vi "GUI_TRA_Staging.vi"() -> ()   [LabVIEW 2013]
uses:
  <vilib>/Utility/file.llb/Write To Spreadsheet File (DBL).vi
  <vilib>/Utility/file.llb/Write To Spreadsheet File (string).vi
  Device Drivers/TRAServer/HomingType_TypDef.ctl
  Device Drivers/TRAServer/TRAServer.lvclass
  Device Drivers/TRAServer/StatusTRA_TypDef.ctl
  Device Drivers/shared/OnOffTypeDef.ctl
panel:
  in  "Multicolumn Listbox 2":refnum<vi>
  in  "Main Tap 2":refnum<vi>
  out "all pos array":refnum<vi>[][](array[refnum])
  out "all status array":refnum<vi>[][](array[refnum])
  out "indecator ref array 2":refnum<vi>[](array[refnum])
  out "indecator ref array":refnum<vi>[](array[refnum])
  in  "time to wait (TCP) 2":i32=10
  in  "plot":bool=TRUE
  out "ratio(h)":bool
  out "fixsize":bool
  out "error (h)":bool
  out "Device Name (h)":string="StagingTRA1"
  in  "Main Tap":T1(tab)
  in  "stepSize":dbl=0.01
  in  "Status":T2=enum."DISABLE" caption="Status Y"
  in  "Up":bool
  in  "Down":bool
  in  "Right":bool
  in  "Left":bool
  in  "Status":T2=enum."DISABLE" caption="Status X"
  in  "Position":dbl caption="X" format="%#_12g"
  in  "Position":dbl caption="Y" format="%#_12g"
  in  "Mirror":T3(ring)=enum."DiagStage"
  in  "device status":string="Initialized"
  in  "Home 3":bool
  in  "Home 2":bool
  out "Status.Axis 6":T2=enum."DISABLE" caption="Status X"
  out "Status.Axis 5":T2=enum."DISABLE" caption="Status X"
  out "Status.Axis 4":T2=enum."DISABLE" caption="Status X"
  out "Status.Axis 3":T2=enum."DISABLE" caption="Status X"
  out "Status.Axis 2":T2=enum."DISABLE" caption="Status X"
  out "Status.Axis 1":T2=enum."DISABLE" caption="Status X"
  out "Status.Axis 1":T2=enum."DISABLE" caption="Status X"
  out "Status.Axis 2":T2=enum."DISABLE" caption="Status X"
  out "Status.Axis 3":T2=enum."DISABLE" caption="Status X"
  out "Status.Axis 4":T2=enum."DISABLE" caption="Status X"
  out "Status.Axis 5":T2=enum."DISABLE" caption="Status X"
  out "Status.Axis 6":T2=enum."DISABLE" caption="Status X"
  out "Status.Axis 7":T2=enum."DISABLE" caption="Status X"
  out "Status.Axis 8":T2=enum."DISABLE" caption="Status X"
  out "Status.Axis 9":T2=enum."DISABLE" caption="Status X"
  out "Status.Axis 10":T2=enum."DISABLE" caption="Status X"
  out "Status.Axis 11":T2=enum."DISABLE" caption="Status X"
  out "Status.Axis 12":T2=enum."DISABLE" caption="Status X"
  in  "Home 1":bool
  in  "Path":path
  in  "Save":bool
  in  "Multicolumn Listbox":i32(listbox)
  in  "Position.Axis 1":dbl=3.05 caption="X"
  in  "Position.Axis 2":dbl=3.05 caption="Y"
  in  "Position.Axis 4":dbl=3.05 caption="X"
  in  "Position.Axis 3":dbl=3.05 caption="Y"
  in  "Position.Axis 6":dbl=3.05 caption="X"
  in  "Position.Axis 5":dbl=3.05 caption="Y"
  in  "Position.Axis 18":dbl=3.05 caption="X"
  in  "Position.Axis 17":dbl=3.05 caption="Y"
  in  "Position.Axis 16":dbl=3.05 caption="X"
  in  "Position.Axis 15":dbl=3.05 caption="Y"
  in  "Position.Axis 14":dbl=3.05 caption="X"
  in  "Position.Axis 13":dbl=3.05 caption="Y"
  in  "Position.Axis 12":dbl=3.05 caption="X"
  in  "Position.Axis 11":dbl=3.05 caption="Y"
  in  "Position.Axis 10":dbl=3.05 caption="X"
  in  "Position.Axis 9":dbl=3.05 caption="Y"
  in  "Position.Axis 8":dbl=3.05 caption="Y"
  in  "Position.Axis 7":dbl=3.05 caption="X"
  in  "take images":bool
  out "appended array 4":cluster{dbl[], dbl[]}[](graph)
  in  "Boolean":bool
  in  "path":path=path "I:/project/Staging/TRAMotors/temp"
  out "centerY":dbl=547.3047962900782
  out "centerX":dbl=832.2888350246396
  in  "backlash":dbl
  in  "backlash 2":dbl
  out "local Port":u16=65435
  in  "timeout ms (slow resp)":i32=500
  in  "reset":bool
  out "image con closed":bool
  out "image \nconnection":bool
  out "image con closed 2":bool
  out "All Devices (h)":string[](array[string])=["StagingTRA1"]
  out "Remote Host":string="192.168.11.97"
  out "port or service name":u16=65434
  out "port or service name out":u16=65400
  in  "time to wait (TCP)":i32=10
  out "error out":errorcluster
  out "connections (hidden)":variant[](array[variant])=[variant(refnum<k16> refnum), variant(refnum<k16> refnum)]
  in  "time to wait (main loop)":i32=10
  out "Data String":string="Status.Axis 1,DISABLE\r\nStatus.Axis 2,DISABLE\r\nStatus.Axis 3,NOT REFERENCED\r\nStatus.Axis 4,NOT REFERENCED\r\nStatus.Axis 5,DISABLE\r\nStatus.Axis 6,NOT REFERENCED\r\nPosition.Axis 1,3.779970\r\nPosition.Axis 2,2.684000\r\nPosition.Axis 3,-0.000000\r\nPosition.Axis 4,-0.000000\r\nPosition.Axis 5,0.000000\r\nPosition.Axis 6,39.383880\r\nDisable.Axis 1,on\r\nDisable.Axis 2,on\r\nDisable.Axis 3,on\r\nDisable.Axis 4,on\r\nDisable.Axis 5,on\r\nDisable.Axis 6,on\r\nHomingType.Axis 1,EoR- switch only\r\nHomingType.Axis 2,EoR- switch only\r\nHomingType.Axis 3,EoR- switch only\r\nHomingType.Axis 4,EoR- switch only\r\nHomingType.Axis 5,MZ switch only\r\nHomingType.Axis 6,EoR- switch only\r\nHome.Axis 1,off\r\nHome.Axis 2,off\r\nHome.Axis 3,off\r\nHome.Axis 4,off\r\nHome.Axis 5,off\r\nHome.Axis 6,off\r\nLimits.pos.Axis 1,6.000000\r\nLimits.pos.Axis 2,6.000000\r\nLimits.pos.Axis 3,6.000000\r\nLimits.pos.Axis 4,6.000000\r\nLimits.pos.Axis 5,51.000000\r\nLimits.pos.Axis 6,6.000000\r\nLimits.neg.Axis 1,0.000000\r\nLimits.neg.Axis 2,0.000000\r\nLimits.neg.Axis 3,0.000000\r\nLimits.neg.Axis 4,0.000000\r\nLimits.neg.Axis 5,-49.000000\r\nLimits.neg.Axis 6,0.000000\r\nbacklash.Axis 1,\r\nbacklash.Axis 2,\r\nbacklash.Axis 3,\r\nbacklash.Axis 4,\r\nbacklash.Axis 5,\r\nbacklash.Axis 6,\r\ndevice status,Initialized\r\n"
  in  "Local Saving Path":path
  out "Nr.":i32=2
  out "error (h) 2":bool
  in  "shotnumber":i32
  out "String":string="wait>>Status.Axis 1,Status.Axis 2,Status.Axis 3,Status.Axis 4,Status.Axis 5,Status.Axis 6,Position.Axis 1,Position.Axis 2,Position.Axis 3,Position.Axis 4,Position.Axis 5,Position.Axis 6,Disable.Axis 1,Disable.Axis 2,Disable.Axis 3,Disable.Axis 4,Disable.Axis 5,Disable.Axis 6,HomingType.Axis 1,HomingType.Axis 2,HomingType.Axis 3,HomingType.Axis 4,HomingType.Axis 5,HomingType.Axis 6,Home.Axis 1,Home.Axis 2,Home.Axis 3,Home.Axis 4,Home.Axis 5,Home.Axis 6,Limits.pos.Axis 1,Limits.pos.Axis 2,Limits.pos.Axis 3,Limits.pos.Axis 4,Limits.pos.Axis 5,Limits.pos.Axis 6,Limits.neg.Axis 1,Limits.neg.Axis 2,Limits.neg.Axis 3,Limits.neg.Axis 4,Limits.neg.Axis 5,Limits.neg.Axis 6,TargetPos.Axis 1,TargetPos.Axis 2,TargetPos.Axis 3,TargetPos.Axis 4,TargetPos.Axis 5,TargetPos.Axis 6,backlash.Axis 1,backlash.Axis 2,backlash.Axis 3,backlash.Axis 4,backlash.Axis 5,backlash.Axis 6,device status"
  in  "Limits.pos":dbl=51.0
  in  "Home":T4
  in  "Disable":T4=enum."on"
  in  "HomingType":T5=enum."MZ switch only"
  in  "Disable":T4=enum."on"
  in  "HomingType":T5=enum."MZ switch only"
  in  "Home":T4
  in  "Limits.pos":dbl=51.0
  in  "Limits.neg":dbl=-49.0
  in  "Limits.neg":dbl=-49.0
  in  "Mirror 2":T3(ring)
  out "error message":string
  out "Data Connection out":bool=TRUE
  # "Position"
  # "Chassi 1"
  # "Chassi 2"
  # "Chassi 3"
  # "X"
  # "Y"
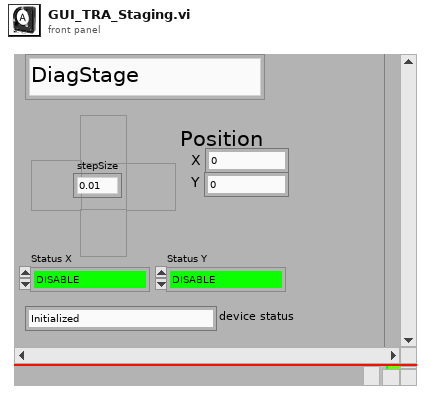
[diagram p1: front panel]
types:
  T1 = enum32{"Main", "Status", "Position", "Position 2", "Temp", "Network", "Internal", "MotorSettings"}
  T2 = typedef "TRAServer.lvclass/StatusTRA_TypDef.ctl" = enum16{"NOT REFERENCED", "CONFIGURATION", "HOMING", "MOVING", "READY", "DISABLE", "JOGGING"}
  T3 = enum16{"M1", "BS", "M3", "OAP1", "M4", "OAP2", "M5", "DiagStage", "SIM"}
  T4 = typedef "OnOffTypeDef.ctl" = enum16{"off", "on"}
  T5 = typedef "TRAServer.lvclass/HomingType_TypDef.ctl" = enum16{"MZ switch and encoder Index", "current position as HOME", "MZ switch only", "EoR- switch and encoder Index", "EoR- switch only"}
  T6 = cluster{"Chassi Nr":i32, "X":string, "Y":string, "name":string}[]
  T7 = cluster{"Chassi Nr":i32, "X":string, "Y":string, "name":string}
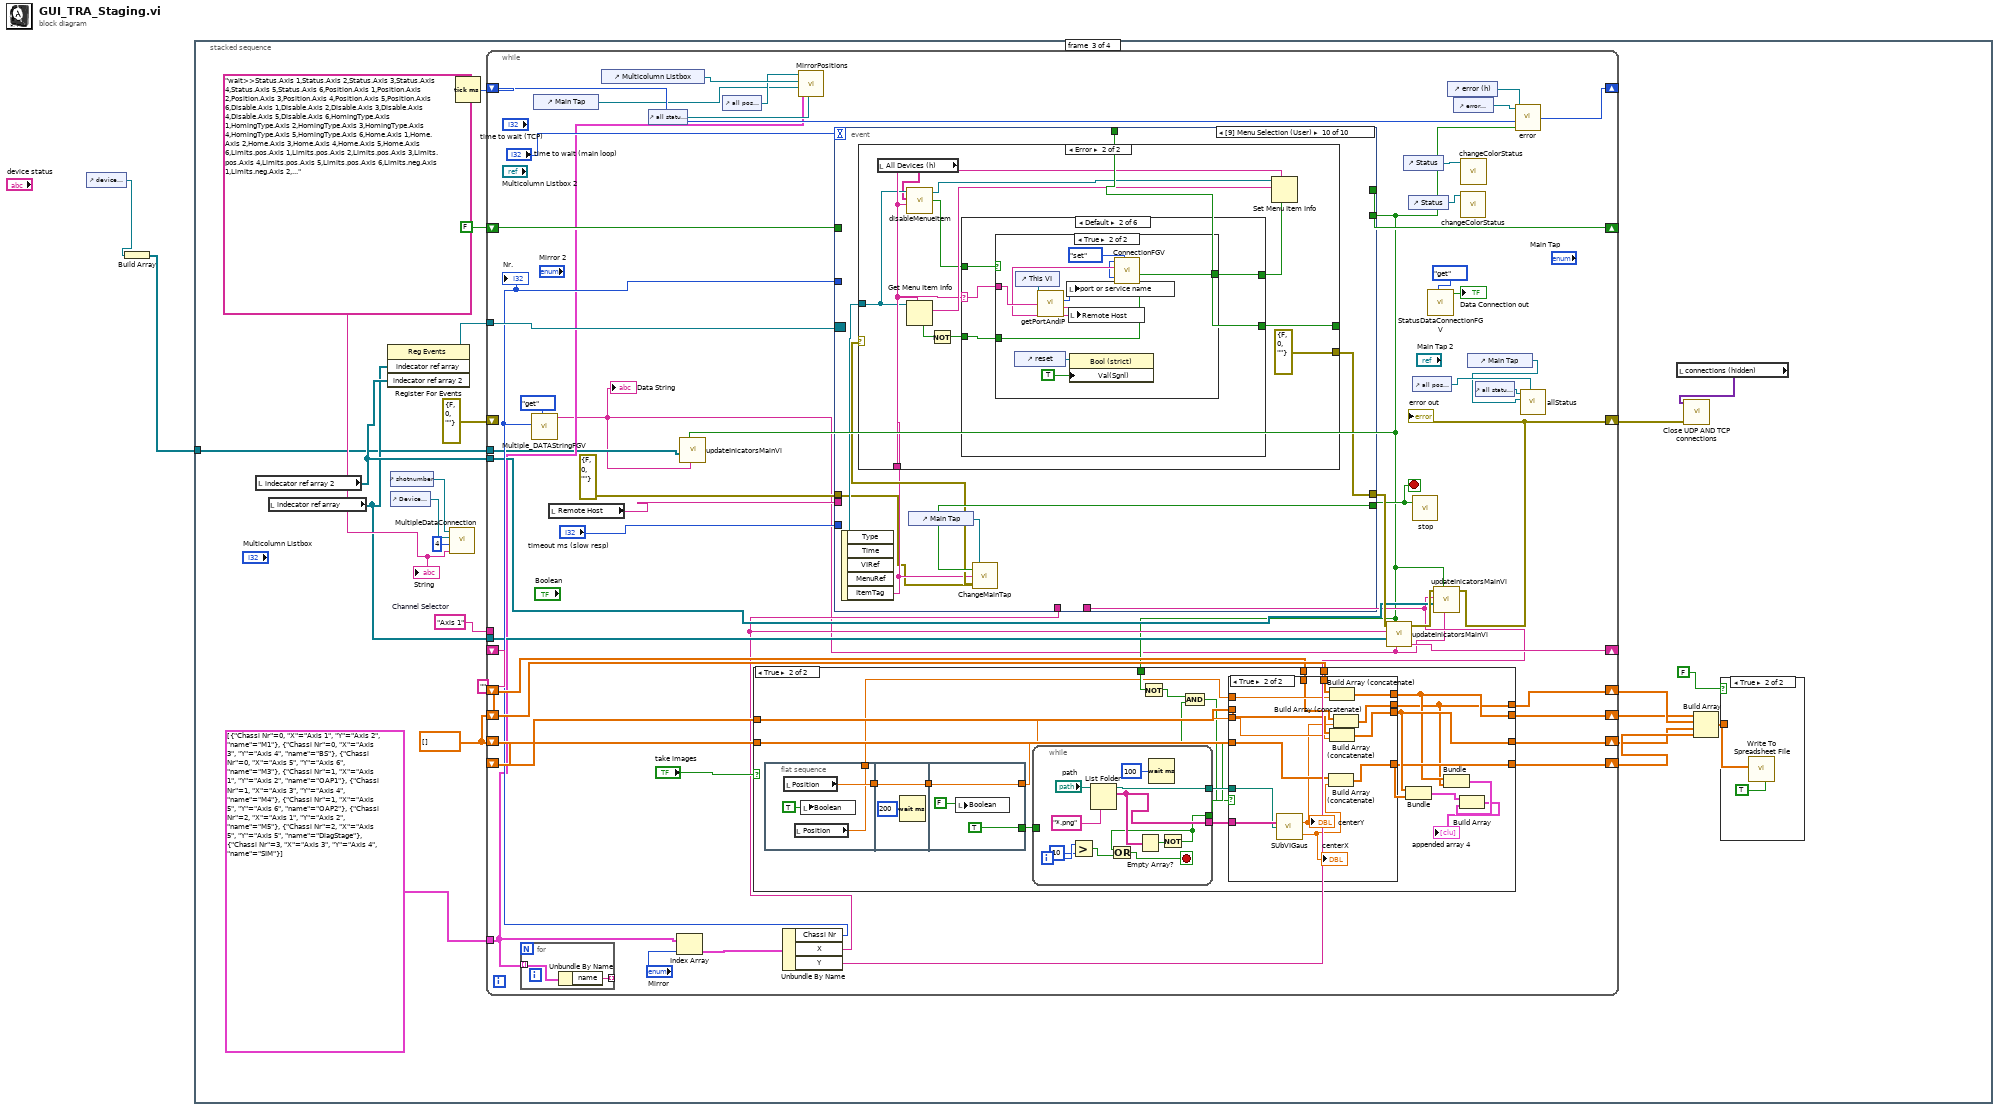
[diagram p0: block diagram]
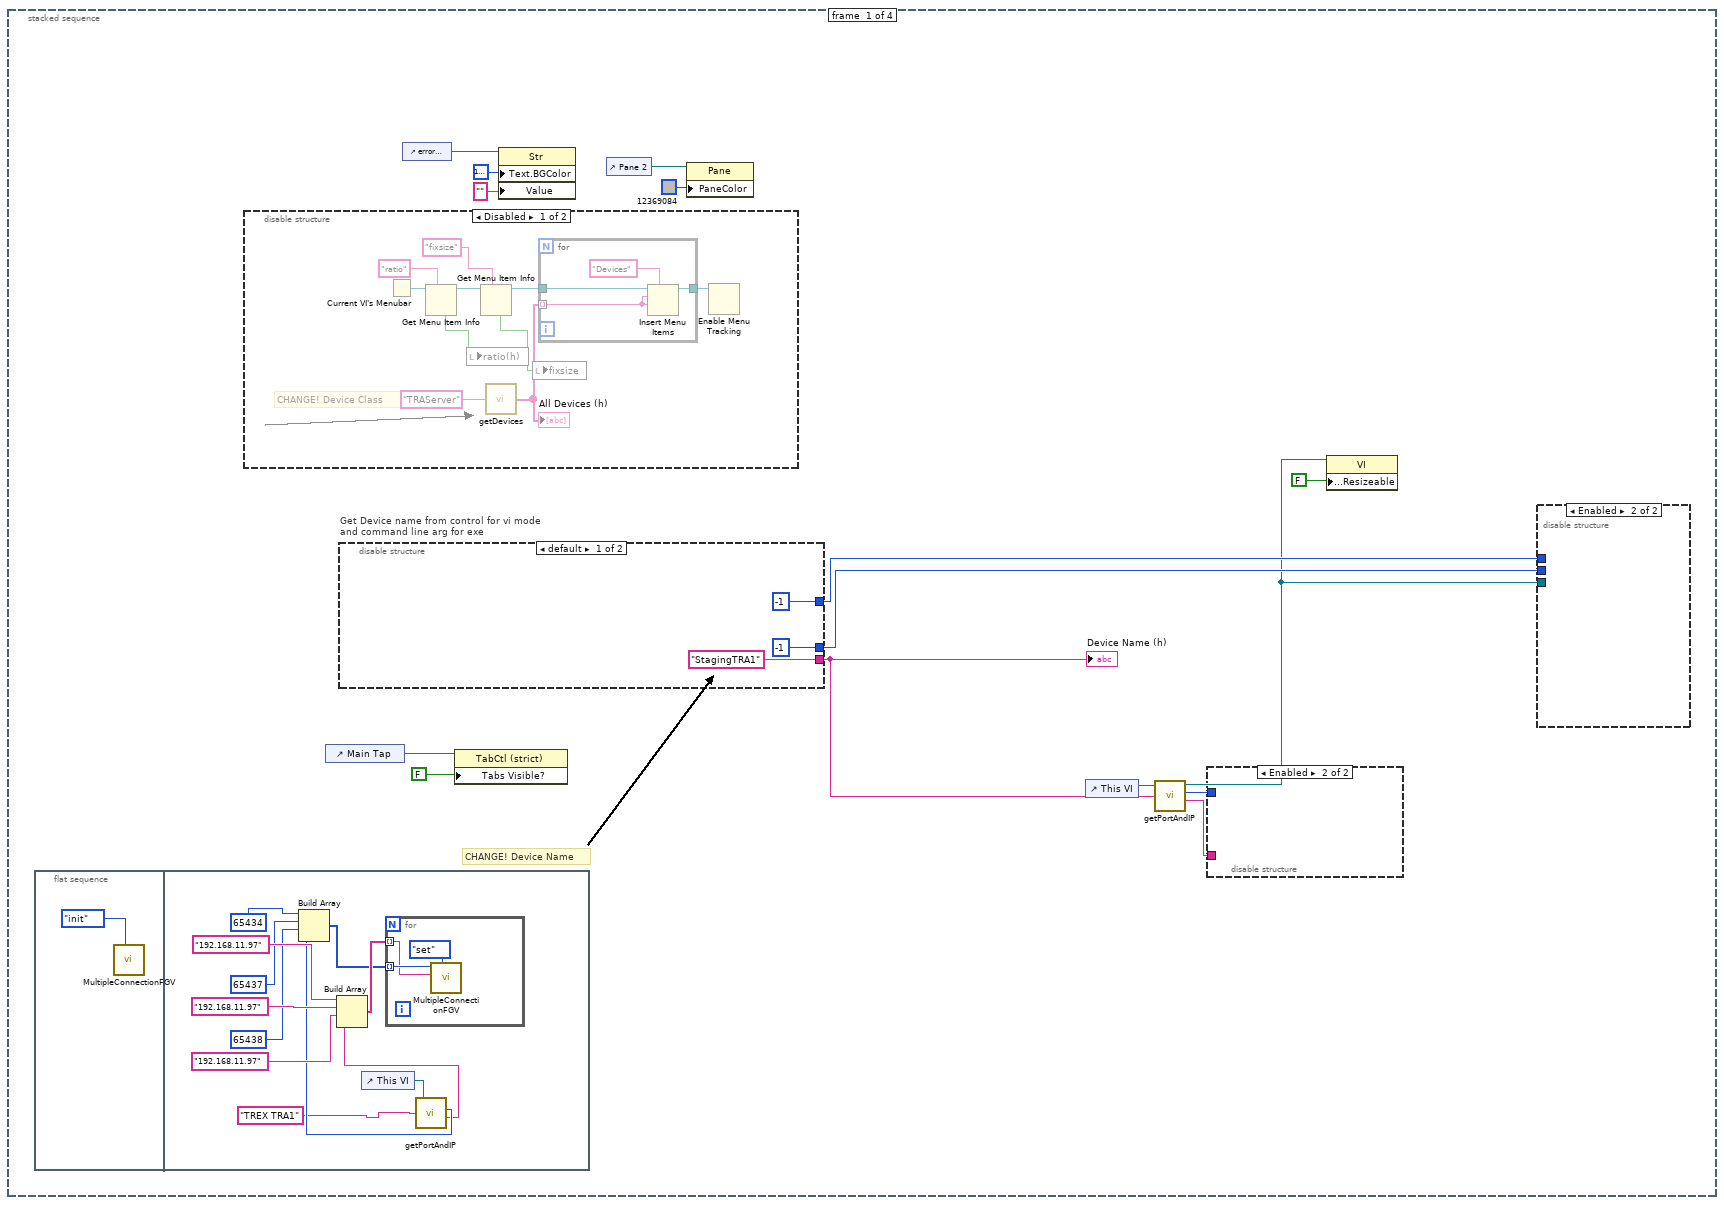
[diagram p2: hidden frame]
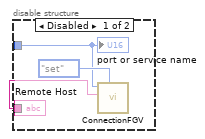
[diagram p4: hidden frame]
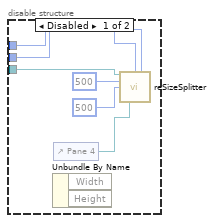
[diagram p5: hidden frame]
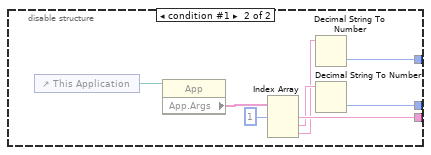
[diagram p6: hidden frame]
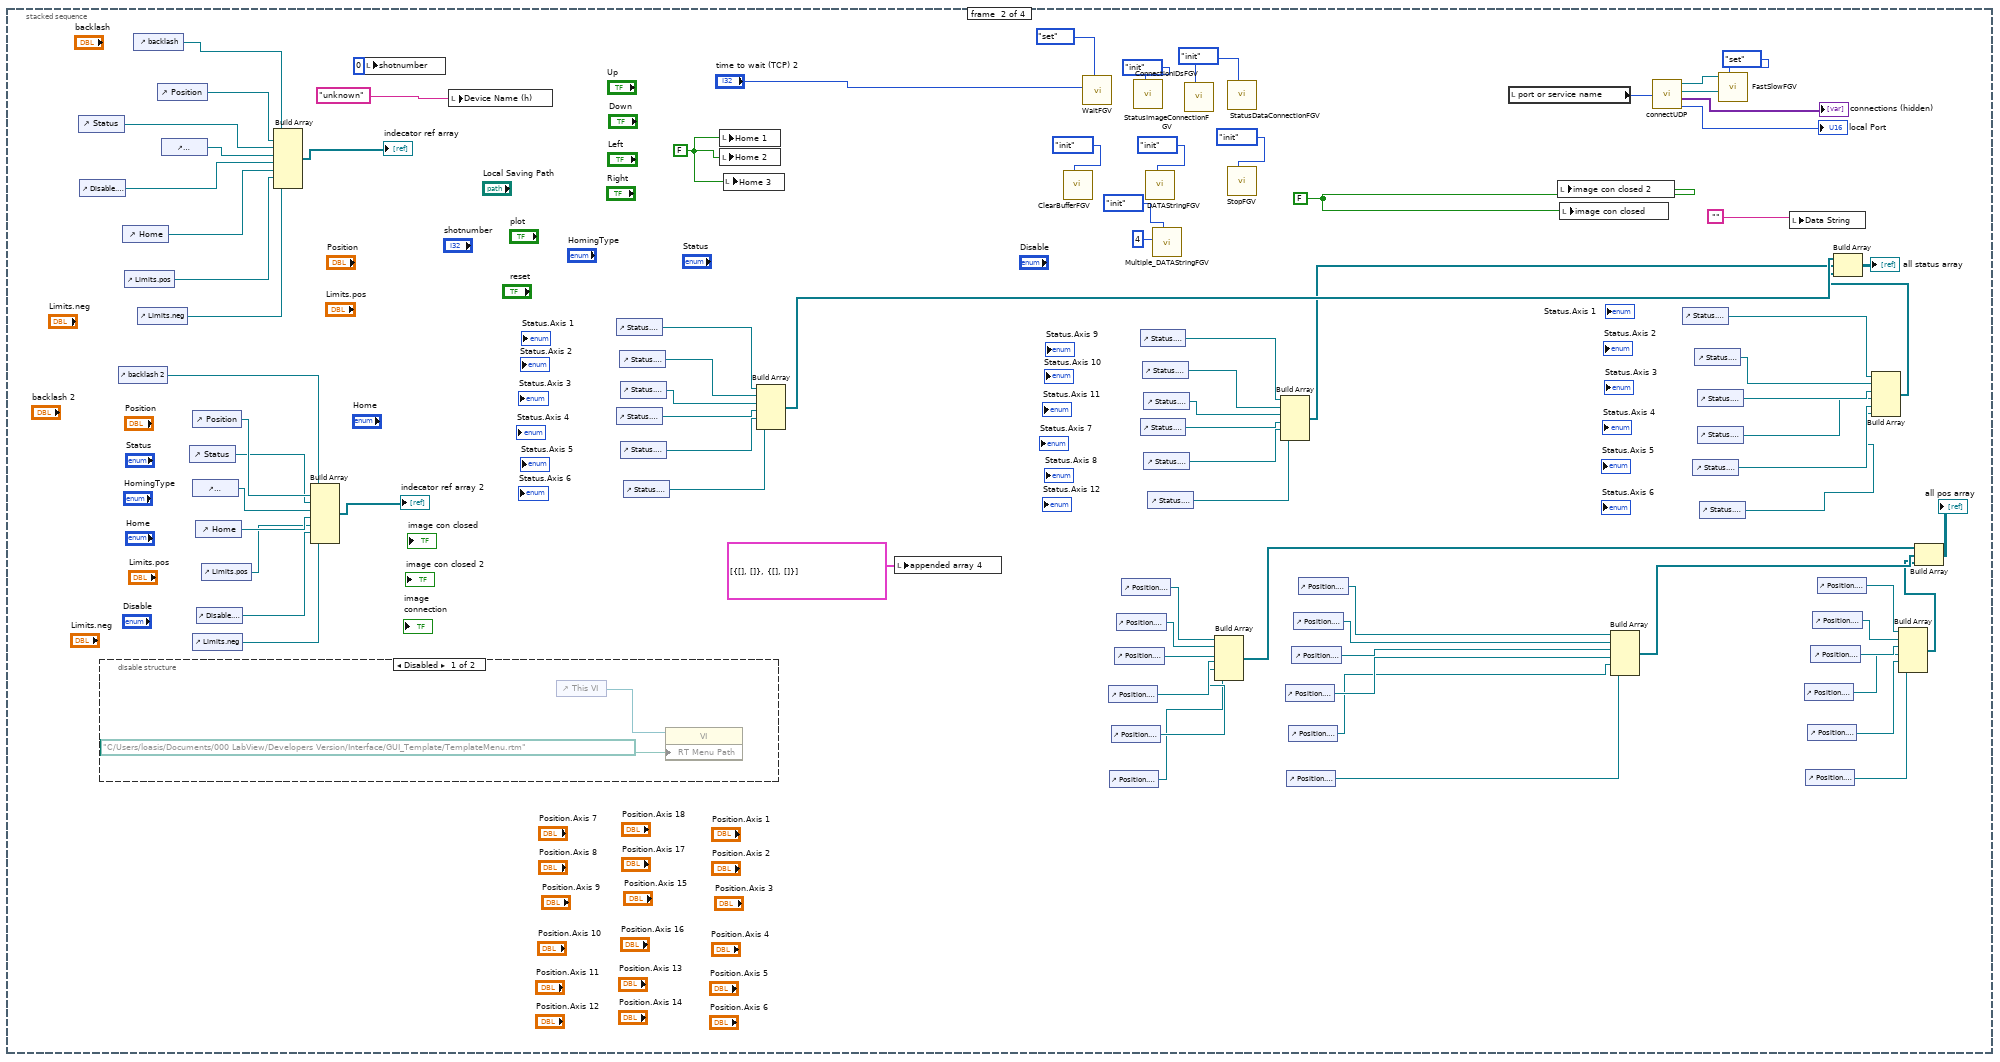
[diagram p7: hidden frame]
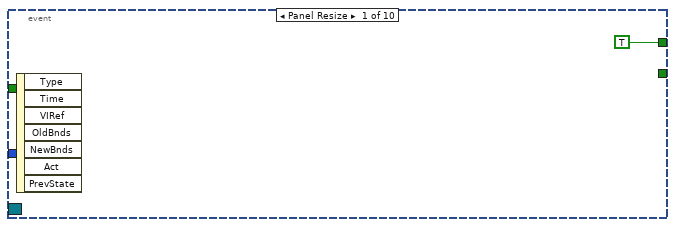
[diagram p12: hidden frame]
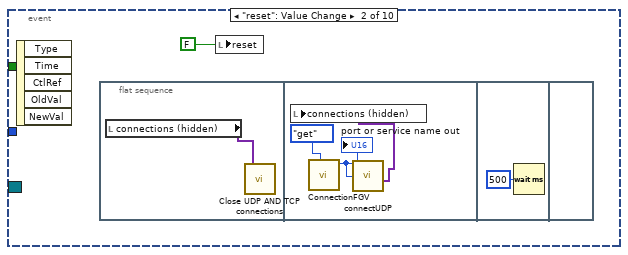
[diagram p13: hidden frame]
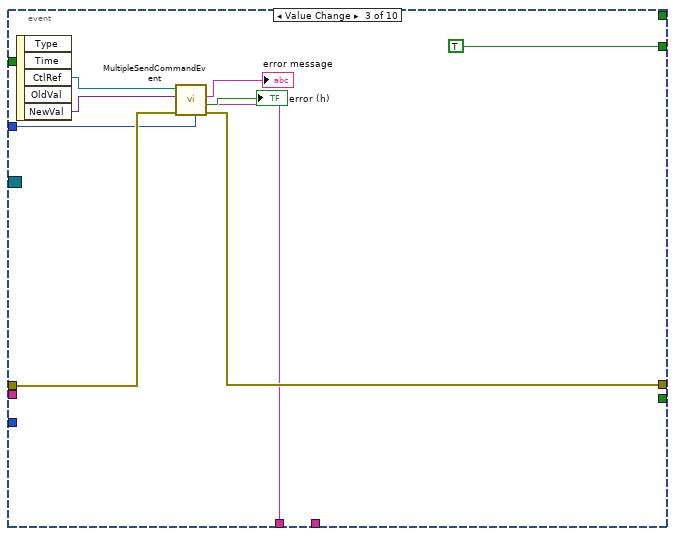
[diagram p14: hidden frame]
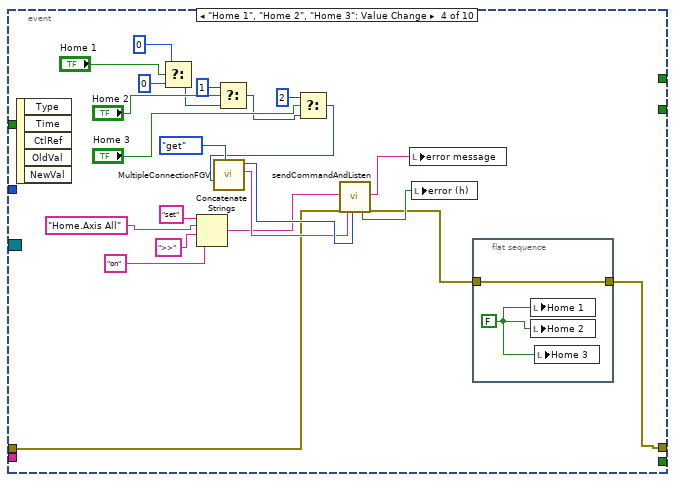
[diagram p15: hidden frame]
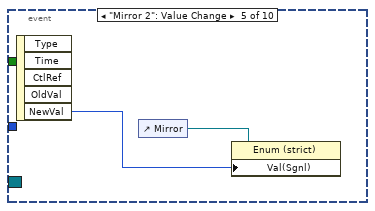
[diagram p16: hidden frame]
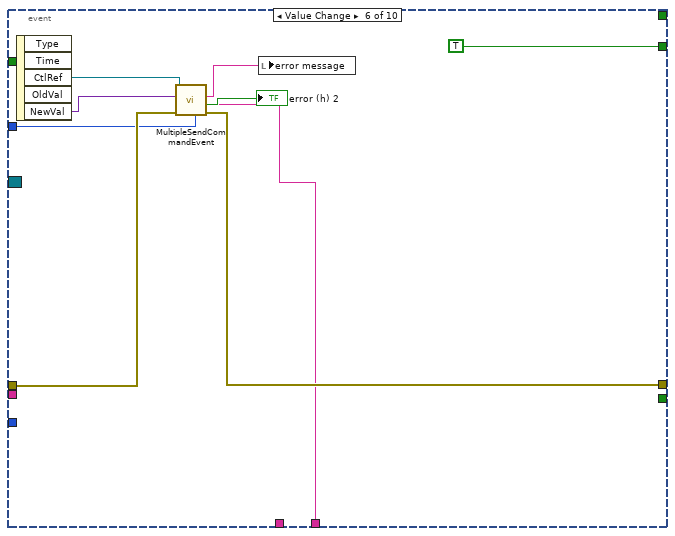
[diagram p17: hidden frame]
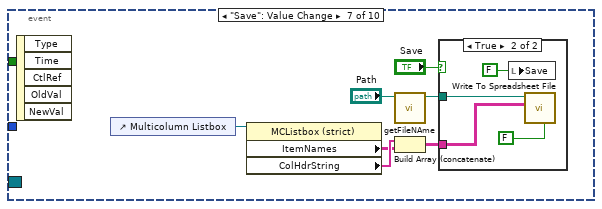
[diagram p18: hidden frame]
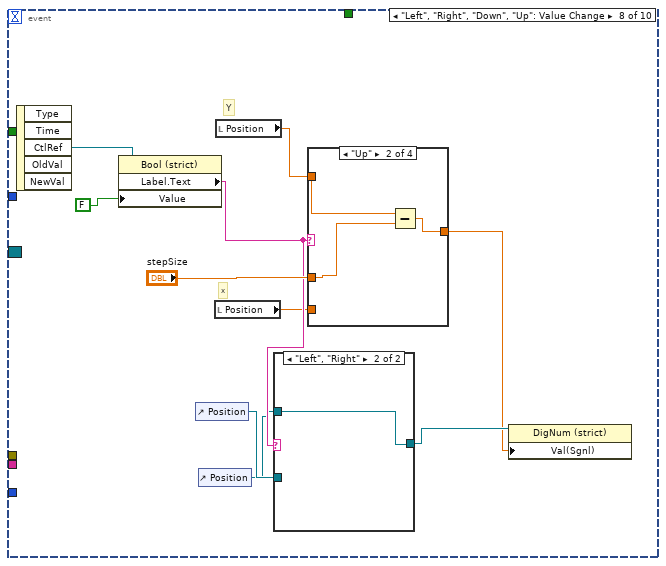
[diagram p20: hidden frame]
diagram:
  n1 = control-ref of="device status"() -> (w2:refnum<vi>)
  n2 = Build Array(w2) -> (w1:refnum<vi>[])
  n3 = stacked-sequence {
    tunnel: w1 -> [_ _ w153 _]
    frame #0 {
      # "CHANGE! Device Name"
      n4 = flat-sequence {
        frame #0 {
          n5 = call "MultipleConnectionFGV.vi"("command"=enum16{"get", "set", "init"}."init") -> ()  [unwired: 9 in, 2 out]
        }
        frame #1 {
          n6 = control-ref of="This VI"() -> (w36:refnum<vi>)
          n7 = call "getPortAndIP.vi"("Device Name"="TREX TRA1", "This Vi"=w36) -> ("Remote Host"=w34:string, "port or service name"=w35:u16)  [unwired: 2 in, 3 out]
          n8 = Build Array(u16 65434 ("port or service name"), u16 65437 ("port or service name"), u16 65438 ("port or service name"), w35) -> (w43:u16[])
          n9 = Build Array("192.168.11.97" ("Remote Host"), "192.168.11.97" ("Remote Host"), "192.168.11.97" ("Remote Host"), w34) -> (w44:string[])
          n10 = for {
            tunnel: w43 -> [w46] mode=indexing
            tunnel: w44 -> [w45] mode=indexing
            n11 = call "MultipleConnectionFGV.vi"("command"=enum16{"get", "set", "init"}."set", "Remote Host in"=w45, "port or service name in"=w46) -> ()  [unwired: 7 in, 2 out]
          }
        }
      }
      n12 = disable-structure shown="Disabled" {
        frame Disabled {
          # "CHANGE! Device Class"
          n13 = Current VI's Menubar() -> (w26:refnum<k9>)
          n14 = Get Menu Item Info(7:"ratio" ("item tag"), 11:w26) -> (3:w24:refnum<k9>, 4:w25:bool)  [unwired: 1 in, 5 out]
          n15 = local write "ratio(h)"(w25) -> ()
          n16 = Get Menu Item Info(7:"fixsize" ("item tag"), 11:w24) -> (3:w21:refnum<k9>, 4:w22:bool)  [unwired: 1 in, 5 out]
          n17 = call "getDevices.vi"("Device Class"="TRAServer") -> ("All Devices"=w19:string[])
          "All Devices (h)" <- w19
          n18 = local write "fixsize"(w22) -> ()
          n19 = for {
            tunnel: w21 -> [w31]
            tunnel: [w30] -> w20
            tunnel: w19 -> [w28] mode=indexing
            n20 = Insert Menu Items(5:"Devices" ("menu tag"), 7:w28, 8:w28, 9:w31) -> (3:w30:refnum<k9>)  [unwired: 2 in, 2 out]
          }
          n21 = Enable Menu Tracking(4:w20) -> ()  [unwired: 2 in, 2 out]
        }
        frame Enabled {
        }
      }
      n22 = control-ref of="Main Tap"() -> (w17:refnum<vi>)
      n23 = disable-structure "Get Device name from control for vi mode\nand command line arg for exe" shown="default" {
        disable-tunnel: ["StagingTRA1" ("Device Name for vi mode") w64] -> w13
        disable-tunnel: [i16 -1 ("left") w61] -> w15
        disable-tunnel: [i16 -1 ("left") w60] -> w14
        frame condition #0 (active) {
        }
        frame condition #1 {
          n24 = control-ref of="This Application"() -> (w67:refnum<vi>)
          n25 = property class="App"(reference=w67) -> ("App.Args"=w66:string[])  [unwired: 1 in, 2 out]
          n26 = Index Array(array=w66, index #1=1 ("index")) -> (element #1=w64:string, element #2=w63:string, element #3=w62:string)  [unwired: 2 in]
          n27 = Decimal String To Number(string=w62) -> (number=w60:i32)  [unwired: 2 in, 1 out]
          n28 = Decimal String To Number(string=w63) -> (number=w61:i32)  [unwired: 2 in, 1 out]
        }
      }
      "Device Name (h)" <- w13
      n29 = control-ref of="error message"() -> (w6:refnum<vi>)
      n30 = property class="TabCtl (strict)"(reference=w17, "Tabs Visible?"=FALSE) -> ()  [unwired: 1 in, 2 out]
      n31 = property class="Str"(reference=w6, "Text.BGColor"=u32 16777238, "Value"="") -> ()  [unwired: 1 in, 2 out]
      n32 = control-ref of="Pane 2"() -> (w4:refnum<vi>)
      n33 = property class="Pane"(reference=w4, "PaneColor"=u32 12369084) -> ()  [unwired: 1 in, 2 out]
      n34 = control-ref of="This VI"() -> (w12:refnum<vi>)
      n35 = call "getPortAndIP.vi"("Device Name"=w13, "This Vi"=w12) -> ("Remote Host"=w9:string, "port or service name"=w8:u16, "reference out"=w10:refnum<vi>)  [unwired: 2 in, 2 out]
      n36 = disable-structure shown="Enabled" {
        disable-tunnel: w9 -> [w49 _]
        disable-tunnel: w8 -> [w48 _]
        frame Disabled {
          n37 = call "ConnectionFGV.vi"("command"=enum16{"get", "set", "init"}."set", "Remote Host in"=w49, "port or service name in"=w48) -> ()  [unwired: 7 in, 2 out]
          "port or service name" <- w48
          "Remote Host" <- w49
        }
        frame Enabled {
        }
      }
      n38 = property class="VI"(reference=w10, "Front Panel.Resizeable"=FALSE ("Front Panel Window:Resizable")) -> ()  [unwired: 1 in, 2 out]
      n39 = disable-structure shown="Enabled" {
        disable-tunnel: w15 -> [w56 _]
        disable-tunnel: w14 -> [w55 _]
        disable-tunnel: w10 -> [w53 _]
        frame Disabled {
          n40 = Unbundle By Name() -> ()  [unwired: 1 in, 2 out]
          n41 = control-ref of="Pane 4"() -> (w54:refnum<vi>)
          n42 = call "reSizeSplitter.vi"("this vi"=w53, "left"=w56, "top"=w55, "Width"=u32 500, "Height"=u32 500, "pane2"=w54) -> ()  [unwired: 9 in, 1 out]
        }
        frame Enabled {
        }
      }
    }
    frame #1 {
      w93 = FALSE
      w142 = enum16{"get", "set", "init"}."init" ("Command")
      w148 = FALSE ("new Device Data")
      n43 = control-ref of="Status"() -> (w131:refnum<vi>)
      n44 = control-ref of="Disable.Axis 1"() -> (w129:refnum<vi>)
      n45 = disable-structure shown="Disabled" {
        frame Disabled {
          n46 = control-ref of="This VI"() -> (w152:refnum<vi>)
          n47 = property class="VI"(reference=w152, "RT Menu Path"=path "C:/Users/loasis/Documents/000 LabView/Developers Version/Interface/GUI_Template/TemplateMenu.rtm" ("Run-Time Menu Path")) -> ()  [unwired: 1 in, 2 out]
        }
        frame Enabled {
        }
      }
      n48 = control-ref of="backlash 2"() -> (w69:refnum<vi>)
      n49 = control-ref of="Home"() -> (w128:refnum<vi>)
      n50 = control-ref of="Limits.pos"() -> (w127:refnum<vi>)
      n51 = control-ref of="backlash"() -> (w68:refnum<vi>)
      n52 = control-ref of="Limits.neg"() -> (w117:refnum<vi>)
      n53 = control-ref of="Position"() -> (w132:refnum<vi>)
      n54 = control-ref of="HomingType.Axis 1"() -> (w130:refnum<vi>)
      n55 = control-ref of="Status"() -> (w123:refnum<vi>)
      n56 = control-ref of="Position"() -> (w124:refnum<vi>)
      n57 = control-ref of="HomingType"() -> (w122:refnum<vi>)
      n58 = control-ref of="Limits.neg"() -> (w116:refnum<vi>)
      n59 = control-ref of="Home"() -> (w121:refnum<vi>)
      n60 = control-ref of="Disable.Axis"() -> (w119:refnum<vi>)
      n61 = control-ref of="Limits.pos"() -> (w120:refnum<vi>)
      n62 = Build Array(w68, w132, w131, w130, w129, w128, w127, w117) -> (→"indecator ref array":refnum<vi>[])
      n63 = Build Array(w69, w124, w123, w122, w121, w120, w119, w116) -> (→"indecator ref array 2":refnum<vi>[])
      n64 = local write "shotnumber"(0 ("shotnumber")) -> ()
      n65 = local write "Device Name (h)"("unknown" ("Device Name")) -> ()
      n66 = control-ref of="Status.Axis 1"() -> (w98:refnum<vi>)
      n67 = control-ref of="Status.Axis 4"() -> (w101:refnum<vi>)
      n68 = control-ref of="Status.Axis 2"() -> (w99:refnum<vi>)
      n69 = control-ref of="Status.Axis 3"() -> (w100:refnum<vi>)
      n70 = control-ref of="Status.Axis 5"() -> (w102:refnum<vi>)
      n71 = control-ref of="Status.Axis 6"() -> (w103:refnum<vi>)
      n72 = local write "Home 1"(w93) -> ()
      n73 = local write "Home 2"(w93) -> ()
      n74 = local write "Home 3"(w93) -> ()
      n75 = Build Array(w98, w99, w100, w101, w102, w103) -> (w97:refnum<vi>[])
      n76 = local write "appended array 4"(cluster{dbl[], dbl[]}[] [{[], []}, {[], []}] ("appended array 4")) -> ()
      n77 = call "ClearBufferFGV.vi"("Command"=enum16{"set", "get", "init"}."init") -> ()  [unwired: 10 in, 1 out]
      n78 = call "WaitFGV.vi"("Command"=enum16{"get", "set", "init"}."set", "milliseconds to wait"="time to wait (TCP) 2") -> ()  [unwired: 9 in, 1 out]
      n79 = control-ref of="Position.Axis 10"() -> (w89:refnum<vi>)
      n80 = control-ref of="Position.Axis 12"() -> (w87:refnum<vi>)
      n81 = control-ref of="Position.Axis 11"() -> (w88:refnum<vi>)
      n82 = control-ref of="Position.Axis 9"() -> (w90:refnum<vi>)
      n83 = control-ref of="Position.Axis 8"() -> (w91:refnum<vi>)
      n84 = control-ref of="Position.Axis 7"() -> (w92:refnum<vi>)
      n85 = call "ConnectionIDsFGV.vi"("Command"=enum16{"add", "get", "init"}."init") -> ()  [unwired: 10 in, 1 out]
      n86 = control-ref of="Status.Axis 9"() -> (w109:refnum<vi>)
      n87 = control-ref of="Status.Axis 7"() -> (w106:refnum<vi>)
      n88 = control-ref of="Status.Axis 10"() -> (w108:refnum<vi>)
      n89 = control-ref of="Status.Axis 11"() -> (w107:refnum<vi>)
      n90 = control-ref of="Status.Axis 8"() -> (w105:refnum<vi>)
      n91 = call "DATAStringFGV.vi"("Command"=enum16{"get", "set", "init"}."init") -> ()  [unwired: 9 in, 2 out]
      n92 = control-ref of="Status.Axis 12"() -> (w104:refnum<vi>)
      n93 = call "Multiple_DATAStringFGV.vi"("Command"=enum16{"get", "set", "init"}."init", "Nr."=4) -> ()  [unwired: 9 in, 1 out]
      n94 = call "StatusImageConnectionFGV.vi"("Command"=w142) -> ()  [unwired: 10 in, 1 out]
      n95 = Build Array(w92, w91, w90, w89, w88, w87) -> (w74:refnum<vi>[])
      n96 = call "StatusDataConnectionFGV.vi"("Command"=w142) -> ()  [unwired: 10 in, 1 out]
      n97 = call "StopFGV.vi"("Command"=enum16{"set", "get", "init"}."init") -> ()  [unwired: 9 in, 2 out]
      n98 = Build Array(w109, w108, w107, w106, w105, w104) -> (w96:refnum<vi>[])
      n99 = control-ref of="Position.Axis 16"() -> (w83:refnum<vi>)
      n100 = control-ref of="Position.Axis 14"() -> (w81:refnum<vi>)
      n101 = control-ref of="Position.Axis 13"() -> (w82:refnum<vi>)
      n102 = control-ref of="Position.Axis 15"() -> (w84:refnum<vi>)
      n103 = control-ref of="Position.Axis 17"() -> (w85:refnum<vi>)
      n104 = control-ref of="Position.Axis 18"() -> (w86:refnum<vi>)
      n105 = local read "port or service name"() -> (w138:u16)
      n106 = local write "image con closed 2"(w148) -> ()
      n107 = local write "image con closed"(w148) -> ()
      n108 = Build Array(w86, w85, w84, w83, w82, w81) -> (w73:refnum<vi>[])
      n109 = call "connectUDP.vi"("port or service name NOT USED"=w138) -> ("fast ID (h)"=w137:refnum<k16>, "slow ID (h)"=w136:refnum<k16>, "connections (hidden)"=→"connections (hidden)":variant[], "local Port"=→"local Port":u16)
      n110 = control-ref of="Status.Axis 1"() -> (w115:refnum<vi>)
      n111 = control-ref of="Status.Axis 5"() -> (w111:refnum<vi>)
      n112 = control-ref of="Status.Axis 2"() -> (w114:refnum<vi>)
      n113 = control-ref of="Status.Axis 3"() -> (w113:refnum<vi>)
      n114 = control-ref of="Status.Axis 4"() -> (w112:refnum<vi>)
      n115 = control-ref of="Status.Axis 6"() -> (w110:refnum<vi>)
      n116 = call "FastSlowFGV.vi"("Command"=enum16{"get", "set", "init"}."set", "slow ID"=w136, "fast ID"=w137) -> ()  [unwired: 7 in, 2 out]
      n117 = local write "Data String"("") -> ()
      n118 = control-ref of="Position.Axis 4"() -> (w77:refnum<vi>)
      n119 = control-ref of="Position.Axis 6"() -> (w75:refnum<vi>)
      n120 = control-ref of="Position.Axis 5"() -> (w76:refnum<vi>)
      n121 = control-ref of="Position.Axis 3"() -> (w78:refnum<vi>)
      n122 = control-ref of="Position.Axis 2"() -> (w79:refnum<vi>)
      n123 = control-ref of="Position.Axis 1"() -> (w80:refnum<vi>)
      n124 = Build Array(w115, w114, w113, w112, w111, w110) -> (w95:refnum<vi>[])
      n125 = Build Array(w97, w96, w95) -> (→"all status array":refnum<vi>[][])
      n126 = Build Array(w80, w79, w78, w77, w76, w75) -> (w72:refnum<vi>[])
      n127 = Build Array(w74, w73, w72) -> (→"all pos array":refnum<vi>[][])
    }
    frame #2 {
      w158 = "wait>>Status.Axis 1,Status.Axis 2,Status.Axis 3,Status.Axis 4,Status.Axis 5,Status.Axis 6,Position.Axis 1,Position.Axis 2,Position.Axis 3,Position.Axis 4,Position.Axis 5,Position.Axis 6,Disable.Axis 1,Disable.Axis 2,Disable.Axis 3,Disable.Axis 4,Disable.Axis 5,Disable.Axis 6,HomingType.Axis 1,HomingType.Axis 2,HomingType.Axis 3,HomingType.Axis 4,HomingType.Axis 5,HomingType.Axis 6,Home.Axis 1,Home.Axis 2,Home.Axis 3,Home.Axis 4,Home.Axis 5,Home.Axis 6,Limits.pos.Axis 1,Limits.pos.Axis 2,Limits.pos.Axis 3,Limits.pos.Axis 4,Limits.pos.Axis 5,Limits.pos.Axis 6,Limits.neg.Axis 1,Limits.neg.Axis 2,Limits.neg.Axis 3,Limits.neg.Axis 4,Limits.neg.Axis 5,Limits.neg.Axis 6,TargetPos.Axis 1,TargetPos.Axis 2,TargetPos.Axis 3,TargetPos.Axis 4,TargetPos.Axis 5,TargetPos.Axis 6,backlash.Axis 1,backlash.Axis 2,backlash.Axis 3,backlash.Axis 4,backlash.Axis 5,backlash.Axis 6,device status" ("String")
      w165 = dbl[] []
      w166 = "Axis 1"  # Channel Selector
      n128 = local read "indecator ref array 2"() -> (w157:refnum<vi>[])
      n129 = local read "indecator ref array"() -> (w156:refnum<vi>[])
      n130 = register-events(w156, w157) -> (reference out=w167:refnum<event-registration>)  [unwired: 2 in, 1 out]
      n131 = control-ref of="shotnumber"() -> (w169:refnum<vi>)
      n132 = control-ref of="Device Name (h)"() -> (w168:refnum<vi>)
      n133 = call "MultipleDataConnection.vi"("Subscriber list 2"=w158, "Nr."=4, "Device Name (h)"=w168, "shotnumber"=w169) -> ()
      n134 = Tick Count (ms)() -> (millisecond timer value=w171:u32)
      n135 = while {
        shift-right: [w199] -> w174
        shift-left: errorcluster {"status"=FALSE, "code"=0, "source"=""} ("error out") -> [_]
        tunnel: w156 -> [w197]
        shift-right: [w220] -> _
        shift-left: FALSE -> [w221]
        shift-right: [w219] -> _
        shift-left: w171 -> [w218]
        shift-right: [w213] -> _
        shift-left: "" ("Data String") -> [_]
        tunnel: w167 -> [w215]
        tunnel: w166 -> [_]
        shift-right: [w208] -> w162
        shift-left: w165 -> [w210]
        shift-right: [w207] -> w163
        shift-left: w165 -> [w209]
        shift-right: [w203] -> w161
        shift-left: w165 -> [w202]
        shift-right: [w205] -> w160
        shift-left: w165 -> [w204]
        tunnel: w157 -> [w196]
        tunnel: T6 [{"Chassi Nr"=0, "X"="Axis 1", "Y"="Axis 2", "name"="M1"}, {"Chassi Nr"=0, "X"="Axis 3", "Y"="Axis 4", "name"="BS"}, {"Chassi Nr"=0, "X"="Axis 5", "Y"="Axis 6", "name"="M3"}, {"Chassi Nr"=1, "X"="Axis 1", "Y"="Axis 2", "name"="OAP1"}, {"Chassi Nr"=1, "X"="Axis 3", "Y"="Axis 4", "name"="M4"}, {"Chassi Nr"=1, "X"="Axis 5", "Y"="Axis 6", "name"="OAP2"}, {"Chassi Nr"=2, "X"="Axis 1", "Y"="Axis 2", "name"="M5"}, {"Chassi Nr"=2, "X"="Axis 5", "Y"="Axis 5", "name"="DiagStage"}, {"Chassi Nr"=3, "X"="Axis 3", "Y"="Axis 4", "name"="SIM"}] -> [w183]
        tunnel: w153 -> [w180]
        stop <- w216 stop-if-true
        n136 = for {
          tunnel: w183 -> [w227] mode=indexing
          tunnel: [w226] -> _ mode=indexing
          n137 = Unbundle By Name(w227) -> ("name"=w226:string)
        }
        n138 = control-ref of="Main Tap"() -> (w181:refnum<vi>)
        n139 = local read "Remote Host"() -> (w223:string)
        n140 = control-ref of="Multicolumn Listbox"() -> (w186:refnum<vi>)
        n141 = control-ref of="all status array"() -> (w184:refnum<vi>)
        n142 = Index Array(array=w183, index="Mirror") -> (element=w187:T7)
        n143 = control-ref of="all pos array"() -> (w185:refnum<vi>)
        n144 = Unbundle By Name(w187) -> ("Chassi Nr"=w198:i32, "X"=w195:string, "Y"=w194:string)
        "Nr." <- w198
        n145 = call "Multiple_DATAStringFGV.vi"("Command"=enum16{"get", "set", "init"}."get", "Nr."=w198) -> ("Data String out"=w178:string)  [unwired: 9 in]
        "Data String" <- w178
        n146 = call "MirrorPositions.vi"("all status array"=w184, "Array"=w183, "reference"=w181, "Multicolumn Listbox 2"=w186, "Array in"=w185) -> ()  [unwired: 7 in]
        n147 = event shown="[9] Menu Selection (User)" {
          selector: w215 -> [_ _ _ _ _ _ _ _ _ _]
          dyn-events: _ -> [_ _ _ _ _ _ _ _ _ _]
          timeout: "time to wait (main loop)" -> [_ _ _ _ _ _ _ _ _ _]
          tunnel: [_ _ w304 w307 _ w340 _ _ w379 w381] -> w222
          tunnel: w223 -> [_ _ _ _ _ _ _ _ _ _]
          tunnel: "timeout ms (slow resp)" -> [_ _ _ _ _ _ _ _ _ _]
          tunnel: errorcluster {"status"=FALSE, "code"=0, "source"=""} ("error out") -> [_ _ w301 w324 _ w338 _ _ w379 w382]
          tunnel: [_ _ TRUE _ _ TRUE _ _ _ _] -> w179
          tunnel: [_ _ _ _ _ _ _ _ _ w387] -> w216
          tunnel: [_ _ _ _ _ _ _ _ w378 w384] -> _
          tunnel: w221 -> [_ _ _ _ _ _ _ _ w378 _]
          tunnel: [TRUE _ _ _ _ _ _ _ _ _] -> w220
          tunnel: w198 -> [_ _ w299 _ _ w336 _ _ _ _]
          tunnel: w195 -> [_ _ w298 _ _ _ _ _ _ _]
          tunnel: w194 -> [_ _ _ _ _ w335 _ _ _ _]
          event Panel Resize {
            n148 = event-data() -> ()  [unwired: 1 in, 7 out]
          }
          event "reset": Value Change {
            n149 = event-data() -> ()  [unwired: 1 in, 5 out]
            n150 = flat-sequence {
              frame #0 {
                n151 = local read "connections (hidden)"() -> (w293:variant[])
                n152 = call "Close UDP AND TCP connections.vi"("appended array"=w293) -> ()  [unwired: 7 in]
              }
              frame #1 {
                n153 = call "ConnectionFGV.vi"("command"=enum16{"get", "set", "init"}."get") -> ("port or service name out"=w295:u16)  [unwired: 9 in, 1 out]
                "port or service name out" <- w295
                n154 = call "connectUDP.vi"("port or service name NOT USED"=w295) -> ("connections (hidden)"=w294:variant[])  [unwired: 3 out]
                n155 = local write "connections (hidden)"(w294) -> ()
              }
              frame #2 {
                n156 = Wait (ms)(milliseconds to wait=u32 500) -> ()  [unwired: 1 out]
              }
              frame #3 {
              }
            }
            n157 = local write "reset"(FALSE ("reset")) -> ()
          }
          event Value Change {
            n158 = event-data() -> ("CtlRef"=w306:refnum<vi>, "NewVal"=w305:variant)  [unwired: 1 in, 3 out]
            n159 = call "MultipleSendCommandEvent.vi"("Nr."=w299, "error out 2"=w301, "Channel Selector"=w298, "NewVal"=w305, "CtlRef"=w306) -> ("error out"=w304:errorcluster, "error (h)"=→"error (h)":bool, "error message"=→"error message":string)  [unwired: 3 in, 1 out]
          }
          event "Home 1", "Home 2", "Home 3": Value Change {
            n160 = event-data() -> ()  [unwired: 1 in, 5 out]
            n161 = Select(t=0 ("Nr."), s="Home 1", f=0) -> (s? t:f=w311:i32)
            n162 = Concatenate Strings("set", "Home.Axis All" ("string"), ">>" ("string"), "on" ("string")) -> (w326:string)
            n163 = Select(t=1 ("Nr."), s="Home 2", f=w311) -> (s? t:f=w312:i32)
            n164 = Select(t=2 ("Nr."), s="Home 3", f=w312) -> (s? t:f=w309:i32)
            n165 = call "MultipleConnectionFGV.vi"("command"=enum16{"get", "set", "init"}."get", "Nr."=w309) -> ("Remote Host out"=w328:string, "port or service name out"=w329:u16)  [unwired: 8 in]
            n166 = call "sendCommandAndListen.vi"("command in"=w326, "error in"=w324, "Remote Host"=w328, "port or service name"=w329) -> ("error"=w322:bool, "error message"=w323:string, "error out"=w308:errorcluster)  [unwired: 8 in, 5 out]
            n167 = local write "error message"(w323) -> ()
            n168 = local write "error (h)"(w322) -> ()
            n169 = flat-sequence {
              tunnel: w308 -> [w331]
              tunnel: [w331] -> w307
              frame #0 {
                w330 = FALSE
                n170 = local write "Home 1"(w330) -> ()
                n171 = local write "Home 2"(w330) -> ()
                n172 = local write "Home 3"(w330) -> ()
              }
            }
          }
          event "Mirror 2": Value Change {
            n173 = event-data() -> ("NewVal"=w332:T3)  [unwired: 1 in, 4 out]
            n174 = control-ref of="Mirror"() -> (w333:refnum<vi>)
            n175 = property class="Enum (strict)"(reference=w333, "Val(Sgnl)"=w332) -> ()  [unwired: 1 in, 2 out]
          }
          event Value Change {
            n176 = event-data() -> ("CtlRef"=w342:refnum<vi>, "NewVal"=w341:variant)  [unwired: 1 in, 3 out]
            n177 = call "MultipleSendCommandEvent.vi"("Nr."=w336, "error out 2"=w338, "Channel Selector"=w335, "NewVal"=w341, "CtlRef"=w342) -> ("error out"=w340:errorcluster, "error (h)"=→"error (h) 2":bool, "error message"=w334:string)  [unwired: 3 in, 1 out]
            n178 = local write "error message"(w334) -> ()
          }
          event "Save": Value Change {
            n179 = event-data() -> ()  [unwired: 1 in, 5 out]
            n180 = control-ref of="Multicolumn Listbox"() -> (w349:refnum<vi>)
            n181 = property class="MCListbox (strict)"(reference=w349) -> ("ItemNames"=w347:string[][], "ColHdrString"=w348:string[])  [unwired: 1 in, 2 out]
            n182 = call "getFileNAme.vi"("Path"="Path") -> ("appended path"=w343:path)  [unwired: 9 in, 1 out]
            n183 = Build Array (concatenate)(w348, w347) -> (w345:string[][])
            n184 = case shown="True" "Save" {
              tunnel: w343 -> [_ w352]
              tunnel: w345 -> [_ w351]
              frame False {
              }
              frame True {
                n185 = local write "Save"(FALSE ("Save")) -> ()
                n186 = call-poly <vilib>:"Write To Spreadsheet File.vi"("transpose? (no:F)"=FALSE, "2D data"=w351, "file path (dialog if empty)"=w352) -> ()  [unwired: 5 in, 1 out]
              }
            }
          }
          event "Left", "Right", "Down", "Up": Value Change {
            # "Y"
            # "x"
            n187 = event-data() -> ("CtlRef"=w363:refnum<vi>)  [unwired: 1 in, 4 out]
            n188 = property class="Bool (strict)"(reference=w363, "Value"=FALSE) -> ("Label.Text"=w360:string)  [unwired: 1 in, 2 out]
            n189 = control-ref of="Position"() -> (w355:refnum<vi>)
            n190 = control-ref of="Position"() -> (w354:refnum<vi>)
            n191 = local read "Position"() -> (w356:dbl)
            n192 = local read "Position"() -> (w361:dbl)
            n193 = case shown="\"Left\", \"Right\"" w360 {
              tunnel: w354 -> [_ w365]
              tunnel: w355 -> [w364 _]
              tunnel: [w364 w365] -> w359
              frame "Down", "Up", Default {
              }
              frame "Left", "Right" {
              }
            }
            n194 = case shown="\"Up\"" w360 {
              tunnel: w356 -> [w367 _ _ w377]
              tunnel: "stepSize" -> [w368 w370 w373 w376]
              tunnel: [w366 w369 w372 w375] -> w358
              tunnel: w361 -> [_ w371 w374 _]
              frame "Right" {
                n195 = Add(x=w368, y=w367) -> (x+y=w366:dbl)
              }
              frame "Up" {
                n196 = Subtract(x=w371, y=w370) -> (x-y=w369:dbl)
              }
              frame "Down", Default {
                n197 = Add(x=w374, y=w373) -> (x+y=w372:dbl)
              }
              frame "Left" {
                n198 = Subtract(x=w377, y=w376) -> (x-y=w375:dbl)
              }
            }
            n199 = property class="DigNum (strict)"(reference=w359, "Val(Sgnl)"=w358) -> ()  [unwired: 1 in, 2 out]
          }
          event Timeout {
            n200 = event-data() -> ()  [unwired: 1 in, 2 out]
          }
          event Menu Selection (User) {
            n201 = event-data() -> ("MenuRef"=w383:refnum<k9>, "ItemTag"=w385:string)  [unwired: 1 in, 3 out]
            n202 = control-ref of="Main Tap"() -> (w380:refnum<vi>)
            n203 = call "ChangeMainTap.vi"("error in"=w382, "ItemTag"=w385, "reference"=w380) -> ("error out"=w386:errorcluster, "Boolean"=w387:bool)
            n204 = case shown="Error" w386 {
              selector: w386 -> [w388 _]
              tunnel: w383 -> [_ w394]
              tunnel: [_ w396] -> w384
              tunnel: w385 -> [_ w395]
              tunnel: [w388 errorcluster {"status"=FALSE, "code"=0, "source"=""} ("error IO")] -> w381
              frame No Error {
              }
              frame Error {
                n205 = local read "All Devices (h)"() -> (w389:string[])
                n206 = call "disableMenueItem.vi"("ItemTag"=w395, "All Devices (h)"=w389, "MenuRef"=w394) -> ("this is a Device(tag)"=w393:bool, "menu reference out"=w392:refnum<k9>)  [unwired: 1 in, 1 out]
                n207 = Get Menu Item Info(7:w395, 11:w394) -> (2:w398:string, 4:w399:bool)  [unwired: 1 in, 5 out]
                n208 = Not(x=w399) -> (.not. x?=w397:bool)
                n209 = case shown="Default" w395 {
                  selector: w395 -> [_ w405 _ _ _ _]
                  tunnel: w397 -> [w400 w403 w415 _ _ _]
                  tunnel: [_ _ TRUE _ _ _] -> w396
                  tunnel: w393 -> [_ w406 _ _ _ _]
                  tunnel: [w400 w404 w415 _ _ _] -> w391
                  frame "fixsize" {
                    n210 = control-ref of="This VI"() -> (w402:refnum<vi>)
                    n211 = Not(x=w400) -> (.not. x?=w401:bool)
                    n212 = property class="VI"(reference=w402, "Front Panel.Resizeable"=w401) -> ()  [unwired: 1 in, 2 out]
                    "fixsize" <- w400
                  }
                  frame Default {
                    n213 = case shown="True" w406 {
                      tunnel: w405 -> [_ w414]
                      tunnel: [_ w410] -> w404
                      tunnel: w403 -> [_ w410]
                      frame False {
                      }
                      frame True {
                        n214 = control-ref of="reset"() -> (w412:refnum<vi>)
                        n215 = control-ref of="This VI"() -> (w413:refnum<vi>)
                        n216 = call "getPortAndIP.vi"("Device Name"=w414, "This Vi"=w413) -> ("Remote Host"=w409:string, "port or service name"=w408:u16)  [unwired: 2 in, 3 out]
                        n217 = local write "port or service name"(w408) -> ()
                        n218 = local write "Remote Host"(w409) -> ()
                        n219 = property class="Bool (strict)"(reference=w412, "Val(Sgnl)"=TRUE ("Value (Signaling)")) -> ()  [unwired: 1 in, 2 out]
                        n220 = call "ConnectionFGV.vi"("command"=enum16{"get", "set", "init"}."set", "Remote Host in"=w409, "port or service name in"=w408) -> ()  [unwired: 7 in, 2 out]
                      }
                    }
                  }
                  frame "ratio" {
                    "ratio(h)" <- w415
                  }
                  frame "Local Saving Path" {
                    n221 = control-ref of="Local Saving Path"() -> (w417:refnum<vi>)
                    n222 = property class="Path"(reference=w417) -> (reference out=w420:refnum<vi>, "Value"=w421:path)  [unwired: 1 in, 1 out]
                    n223 = call "changePath.vi"("Local Saving in (h)"=w421) -> ("change (h)"=w419:bool, "Local Saving out (h)"=w418:path)  [unwired: 9 in]
                    n224 = case shown="True" w419 {
                      tunnel: w420 -> [_ w423]
                      tunnel: w418 -> [_ w422]
                      frame False {
                      }
                      frame True {
                        n225 = property class="Path"(reference=w423, "Val(Sgnl)"=w422) -> ()  [unwired: 1 in, 2 out]
                      }
                    }
                  }
                  frame "reset" {
                    n226 = control-ref of="reset"() -> (w425:refnum<vi>)
                    n227 = property class="Bool (strict)"(reference=w425, "Val(Sgnl)"=TRUE ("Value (Signaling)")) -> ()  [unwired: 1 in, 2 out]
                  }
                  frame "clear" {
                    n228 = control-ref of="reset"() -> (w427:refnum<vi>)
                    n229 = property class="Bool (strict)"(reference=w427, "Val(Sgnl)"=TRUE ("Value (Signaling)")) -> ()  [unwired: 1 in, 2 out]
                  }
                }
                n230 = Set Menu Item Info(6:w391, 7:w395, 10:w398, 11:w392) -> ()  [unwired: 3 in, 2 out]
              }
            }
          }
        }
        n231 = call "updateInicatorsMainVi.vi"("Data String out"=w178, "Boolean"=w179, "Array"=w180) -> ()  [unwired: 6 in, 3 out]
        n232 = case shown="True" "take images" {
          tunnel: w210 -> [w231 w248]
          tunnel: w209 -> [w230 w247]
          tunnel: [w231 w246] -> w208
          tunnel: [w230 w245] -> w207
          tunnel: w179 -> [_ w241]
          tunnel: [w229 w236] -> w205
          tunnel: w204 -> [w229 w238]
          tunnel: [w228 w235] -> w203
          tunnel: w202 -> [w228 w237]
          frame False {
          }
          frame True {
            n233 = flat-sequence {
              tunnel: [w284] -> w253
              tunnel: [w283] -> w239
              tunnel: [w286] -> w252
              tunnel: w253 -> [w286]
              tunnel: [TRUE] -> w249
              tunnel: [w288] -> w244
              tunnel: w252 -> [w288]
              frame #0 {
                n234 = local read "Position"() -> (w284:dbl)
                n235 = local read "Position"() -> (w283:dbl)
                n236 = local write "Boolean"(TRUE ("Boolean")) -> ()
              }
              frame #1 {
                n237 = Wait (ms)(milliseconds to wait=u32 200) -> ()  [unwired: 1 out]
              }
              frame #2 {
                n238 = local write "Boolean"(FALSE ("Boolean")) -> ()
              }
            }
            n239 = while {
              tunnel: [w275] -> w251
              tunnel: [w274] -> w250
              tunnel: w249 -> [_]
              tunnel: [w272] -> w243
              i -> [w278]
              stop <- w279 stop-if-true
              n240 = Greater?(x=w278, y=10) -> (0:w273:bool)
              n241 = List Folder(path="path", pattern="*.png") -> (path out=w274:path, filenames=w275:string[])  [unwired: 2 in, 2 out]
              n242 = Empty Array?(array=w275) -> (empty?=w280:bool)
              n243 = Wait (ms)(milliseconds to wait=u32 100) -> ()  [unwired: 1 out]
              n244 = Not(x=w280) -> (.not. x?=w272:bool)
              n245 = Or(x=w272, y=w273) -> (x .or. y?=w279:bool)
            }
            n246 = Not(x=w241) -> (.not. x?=w242:bool)
            n247 = And(x=w242, y=w243) -> (x .and. y?=w240:bool)
            n248 = case shown="True" w240 {
              tunnel: w251 -> [_ w271]
              tunnel: w250 -> [_ w270]
              tunnel: [w256 w269] -> w246
              tunnel: w248 -> [w256 w268]
              tunnel: [w257 w267] -> w245
              tunnel: w247 -> [w257 w266]
              tunnel: w244 -> [_ w264]
              tunnel: w239 -> [_ w263]
              tunnel: [w254 w261] -> w236
              tunnel: w238 -> [w254 w262]
              tunnel: [w255 w259] -> w235
              tunnel: w237 -> [w255 w258]
              frame False {
              }
              frame True {
                n249 = call "SUbVIGaus.vi"("filenames"=w271, "path out"=w270) -> ("centerX"=w260:dbl, "centerY"=w265:dbl)  [unwired: 5 in, 7 out]
                "centerY" <- w260
                "centerX" <- w265
                n250 = Build Array (concatenate)(w266, w265) -> (w267:dbl[])
                n251 = Build Array (concatenate)(w262, w263) -> (w261:dbl[])
                n252 = Build Array (concatenate)(w268, w264) -> (w269:dbl[])
                n253 = Build Array (concatenate)(w258, w260) -> (w259:dbl[])
              }
            }
            n254 = Bundle(w246, w245) -> (w234:cluster{dbl[], dbl[]})  [unwired: 1 in]
            n255 = Bundle(w236, w235) -> (w233:cluster{dbl[], dbl[]})  [unwired: 1 in]
            n256 = Build Array(w234, w233) -> (→"appended array 4":cluster{dbl[], dbl[]}[])
          }
        }
        n257 = call "updateInicatorsMainVi.vi"("Data String out"=w178, "Boolean"=w179, "Array"=w197, "Channel Selector"=w195, "error in"=w222) -> ("Data String out 2"=w213:string, "error out"=w200:errorcluster)  [unwired: 4 in, 1 out]
        n258 = control-ref of="Status"() -> (w193:refnum<vi>)
        n259 = control-ref of="Status"() -> (w192:refnum<vi>)
        n260 = control-ref of="all pos array"() -> (w188:refnum<vi>)
        n261 = call "stop.vi"("Boolean"=w216) -> ()
        n262 = call "StatusDataConnectionFGV.vi"("Command"=enum16{"get", "set", "init"}."get") -> ("Data Connection out"=→"Data Connection out":bool)  [unwired: 10 in]
        n263 = call "updateInicatorsMainVi.vi"("Data String out"=w178, "Boolean"=w179, "Array"=w196, "Channel Selector"=w194, "error in"=w200) -> ("error out"=w199:errorcluster)  [unwired: 4 in, 2 out]
        "error out" <- w199
        n264 = control-ref of="error (h)"() -> (w211:refnum<vi>)
        n265 = control-ref of="error message"() -> (w212:refnum<vi>)
        n266 = call "changeColorStatus.vi"("Enum in"=w192) -> ()  [unwired: 11 in]
        n267 = call "changeColorStatus.vi"("Enum in"=w193) -> ()  [unwired: 11 in]
        n268 = control-ref of="Main Tap"() -> (w182:refnum<vi>)
        n269 = control-ref of="all status array"() -> (w189:refnum<vi>)
        n270 = call "error.vi"("Boolean"=w179, "millisecond timer value"=w218, "reference"=w211, "error message"=w212) -> ("millisecond timer value 2"=w219:u32)
        n271 = call "allStatus.vi"("all pos array 2"=w188, "generic class reference"=w182, "Array in"=w189) -> ()  [unwired: 9 in]
      }
      n272 = local read "connections (hidden)"() -> (w173:variant[])
      n273 = call "Close UDP AND TCP connections.vi"("error in"=w174, "appended array"=w173) -> ()  [unwired: 6 in]
      n274 = Build Array(w160, w161, w162, w163) -> (w164:dbl[][])
      n275 = case shown="True" FALSE {
        tunnel: w164 -> [_ w177]
        frame False {
        }
        frame True {
          n276 = call-poly <vilib>:"Write To Spreadsheet File.vi"("transpose? (no:F)"=TRUE, "2D data"=w177) -> ()  [unwired: 6 in, 1 out]
        }
      }
      "String" <- w158
    }
    frame #3 {
      n277 = control-ref of="Main  Control"() -> (w429:refnum<vi>)
      n278 = property class="TabCtl (strict)"(reference=w429, "Tabs Visible?"=TRUE) -> ()  [unwired: 1 in, 2 out]
      n279 = property class="TabCtl (strict)"(reference=w429, "Tab Location"=enum32{"Top", "Bottom", "Left", "Right"}."Bottom") -> ()  [unwired: 1 in, 2 out]
      n280 = flat-sequence {
        frame #0 {
          n281 = Wait (ms)(milliseconds to wait=u32 0) -> ()  [unwired: 1 out]
        }
        frame #1 {
        }
        frame #2 {
          n282 = control-ref of="This VI"() -> (w434:refnum<vi>)
          n283 = case shown="True" FALSE {
            tunnel: w434 -> [w435 w438]
            tunnel: [w435 w436] -> w433
            frame False {
            }
            frame True {
              n284 = property class="VI" props=["Front Panel.Open"](reference=w438) -> (reference out=w437:refnum<vi>)  [unwired: 1 in, 2 out]
              n285 = invoke class="VI" method="FP.Close"(reference=w437) -> (reference out=w436:refnum<vi>)  [unwired: 2 in, 2 out]
            }
          }
          n286 = Close Reference(reference=w433) -> ()  [unwired: 1 in, 1 out]
        }
      }
    }
  }
